vi "E02_EstructuraWhile.vi"() -> ()   [LabVIEW 2026]
panel:
  out "Waveform Chart":dbl(graph)
  in  "stop":bool
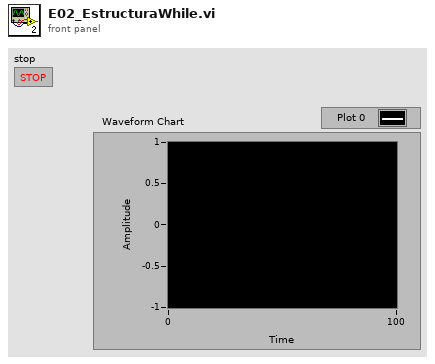
[diagram p1: front panel]
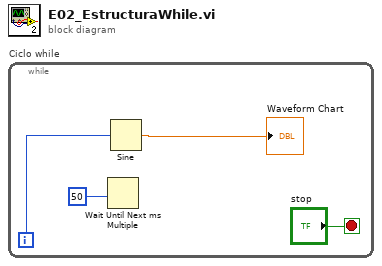
[diagram p0: block diagram]
diagram:
  n1 = while "Ciclo while" {
    i -> [w3]
    stop <- "stop" stop-if-true
    n2 = Wait Until Next ms Multiple(millisecond multiple=50) -> ()  [unwired: 1 out]
    n3 = Sine(x=w3) -> (sin(x)=→"Waveform Chart":dbl)
  }
